vi "Iterate.vi"(10 "Iteration Attempts":u16, 11 "Pixel In":refnum<class "Pixel.lvclass">) -> (3 "Pixel Outs":refnum<class "Pixel.lvclass">)   [LabVIEW 2016, in "Pixel.lvclass"]
uses:
  Pixel.lvclass
  Pixel.lvclass/Pixel.ctl
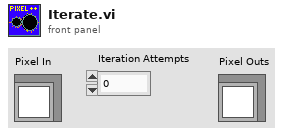
[diagram p1: front panel]
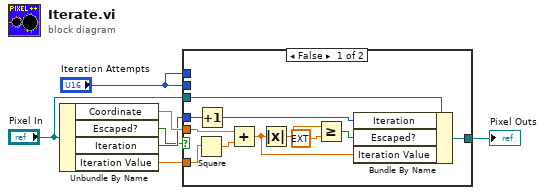
[diagram p0: block diagram]
diagram:
  n1 = Unbundle By Name("Pixel In") -> ("Coordinate"=w7:cdb, "Escaped?"=w4:bool, "Iteration"=w5:u16, "Iteration Value"=w1:cdb)
  n2 = case shown="False" w4 {
    tunnel: w7 -> [w12 _]
    tunnel: "Iteration Attempts" -> [_ _]
    tunnel: "Pixel In" -> [w18 w19]
    tunnel: w5 -> [w11 _]
    tunnel: [w17 w19] -> w3
    tunnel: "Iteration Attempts" -> [_ _]
    tunnel: w1 -> [w13 _]
    frame False {
      n3 = Square(x=w13) -> (x^2=w16:cdb)
      n4 = Increment(x=w11) -> (x+1=w10:u16)
      n5 = Add(x=w12, y=w16) -> (x+y=w9:cdb)
      n6 = Absolute Value(x=w9) -> (abs(x)=w14:dbl)
      n7 = Greater Or Equal?(x=w14, y=ext 2.0) -> (x >= y?=w8:bool)
      n8 = Bundle By Name(cluster=w18, "Iteration"=w10, "Escaped?"=w8, "Iteration Value"=w9) -> (w17:refnum<class "Pixel.lvclass">)
    }
    frame True {
    }
  }
  "Pixel Outs" <- w3
